vi "ArmGetLEDemand.vi"() -> (1 "ExtendPositonDemand(in)":dbl, 2 "LiftPositionDemand(d)":dbl)   [LabVIEW 2020]
doc: "Get postion demand for arm from global varibles\nOutputs:\n--RotatePostionDemand(d)--double--degrees--\n--LiftPostionDemand(d)--double--degrees--\n--ExtendPostionDemand(in)--double--inches--"
uses:
  ArmGlobal.vi
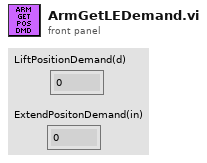
[diagram p1: front panel]
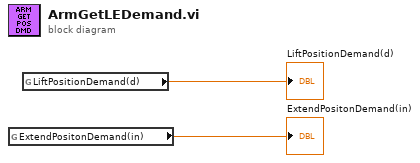
[diagram p0: block diagram]
diagram:
  n1 = global read "ArmGlobal.vi" "ExtendPositonDemand(in)"() -> (→"ExtendPositonDemand(in)":dbl)
  n2 = global read "ArmGlobal.vi" "LiftPositionDemand(d)"() -> (→"LiftPositionDemand(d)":dbl)
